vi "lesstrivial.vi"() -> ()   [LabVIEW 2009]
panel:
  in  "stop":bool
  out "x*x":dbl
  out "sqrt(x)":dbl
  in  "x":dbl
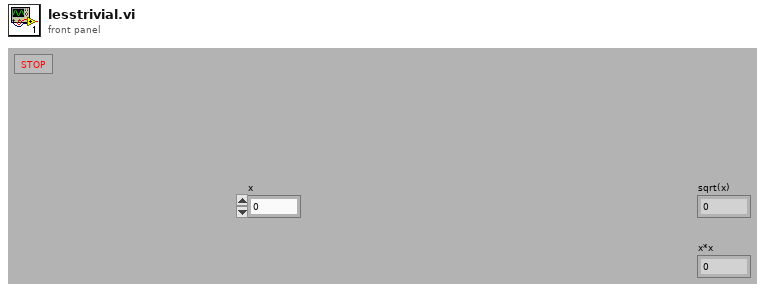
[diagram p1: front panel]
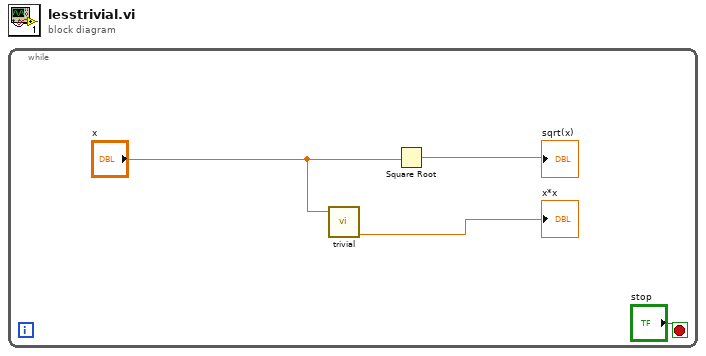
[diagram p0: block diagram]
diagram:
  n1 = while {
    stop <- "stop" stop-if-true
    n2 = call "trivial.vi"("IN"="x") -> ("OUT"=→"x*x":dbl)  [unwired: 10 in]
    n3 = Square Root(x="x") -> (sqrt(x)=→"sqrt(x)":dbl)
  }
